vi "TimeConversions (SubVI).vi"(9 "Ignore Minutes and Seconds":bool, 10 "Current time":i64, 11 "HrToUpdate":i64) -> (1 "Delay_cont":bool, 2 "Time in 64 Bits":i64, 3 "Boolean":bool)   [LabVIEW 2013]
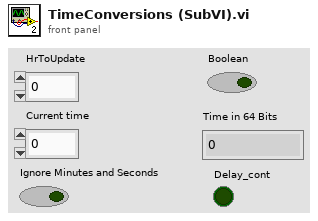
[diagram p1: front panel]
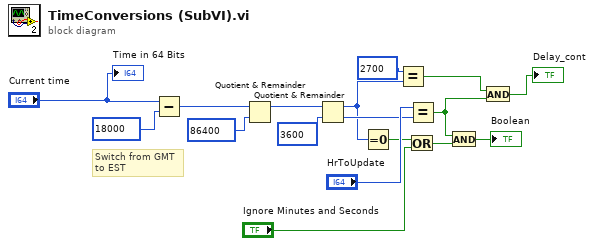
[diagram p0: block diagram]
diagram:
  # "Switch from GMT\nto EST"
  n1 = Subtract(x="Current time", y=i64 18000) -> (x-y=w9:i64)
  n2 = Quotient & Remainder(x=w9, y=i64 86400) -> (x-y*floor(x/y)=w10:i64)  [unwired: 1 out]
  n3 = Quotient & Remainder(x=w10, y=i64 3600) -> (x-y*floor(x/y)=w5:i64, floor(x/y)=w16:i64)
  n4 = Equal To 0?(x=w5) -> (x = 0?=w13:bool)
  n5 = Equal?(x=i64 2700, y=w5) -> (x = y?=w3:bool)
  n6 = Or(x=w13, y="Ignore Minutes and Seconds") -> (x .or. y?=w14:bool)
  n7 = Equal?(x="HrToUpdate", y=w16) -> (x = y?=w1:bool)
  n8 = And(x=w1, y=w14) -> (x .and. y?=→"Boolean":bool)
  n9 = And(x=w3, y=w1) -> (x .and. y?=→"Delay_cont":bool)
  "Time in 64 Bits" <- "Current time"
